vi "Boolean Changed.vi"(7 "error in (no error)":errorcluster, 10 "Boolean in":bool) -> (0 "error in (no error) 2":errorcluster, 2 "Value":bool, 3 "Changed?":bool)   [LabVIEW 2024]
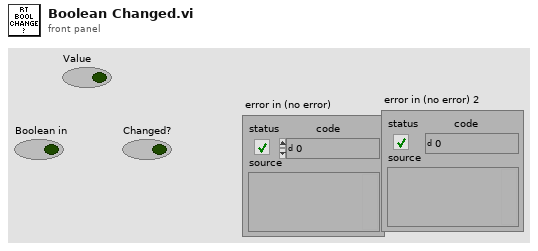
[diagram p1: front panel]
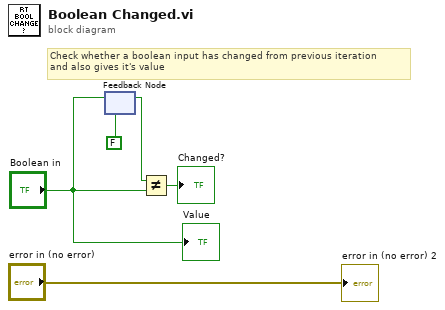
[diagram p0: block diagram]
diagram:
  # "Check whether a boolean input has changed from previous iteration\nand also gives it's value"
  n1 = feedback #1(FALSE ("Boolean")) -> (w2:bool)
  n2 = feedback-in #1("Boolean in") -> ()
  n3 = Not Equal?(x=w2, y="Boolean in") -> (x != y?=→"Changed?":bool)
  "Value" <- "Boolean in"
  "error in (no error) 2" <- "error in (no error)"
